vi "FringeTrackerGUI.vi"() -> ()   [LabVIEW 2009, in "FringeTracker.lvlib"]
uses:
  FringeTracker.lvlib
  Controls/FringeTrackerInfo.ctl
  Nicmos/Controls/NICMOS.READOUT.ctl
  Controls/FringeTrackerData.ctl
panel:
  in  "Autcollimation":bool
  in  "Wavelength":dbl[unit]
  in  "Readout":T1
  out "FringeTrackerInfo":T2={"Readout"={"Readout"=100, "Deglitch"=10, "Framerate"=200.0, "Bank"=2}, "OPD stroke"=0.0, "OPD per pixel"=0.0}
  in  "IDLE Button":bool
  in  "SCAN Button":bool
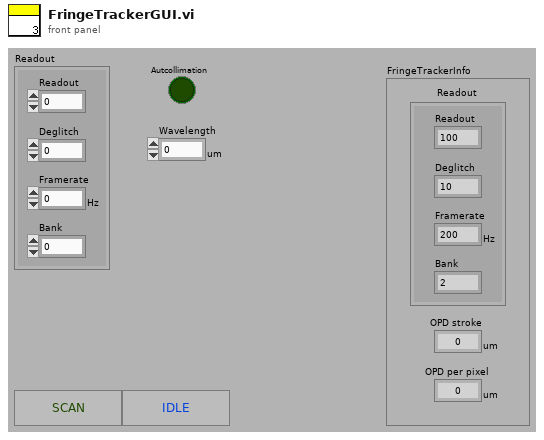
[diagram p1: front panel]
types:
  T1 = typedef "NICMOS.READOUT.ctl" = cluster{"Readout":i32, "Deglitch":i32, "Framerate":dbl[unit], "Bank":i32}
  T2 = typedef "FringeTrackerInfo.ctl" = cluster{"Readout":T1, "OPD stroke":dbl[unit], "OPD per pixel":dbl[unit]}
  T3 = typedef "FringeTrackerData.ctl" = cluster{"Readout":T1, "Wavelength":dbl[unit], "Frame per fringe":dbl, "Autcollimation":bool, "OPD stroke":dbl[unit], "OPD per pixel":dbl[unit], "Offset":dbl[unit]}
  T4 = typedef "FringeTrackerState.ctl" = enum16{"IDLING", "CONFIGURING", "SCANNING", "SEARCHING", "TRACKING", "STOPPING"}
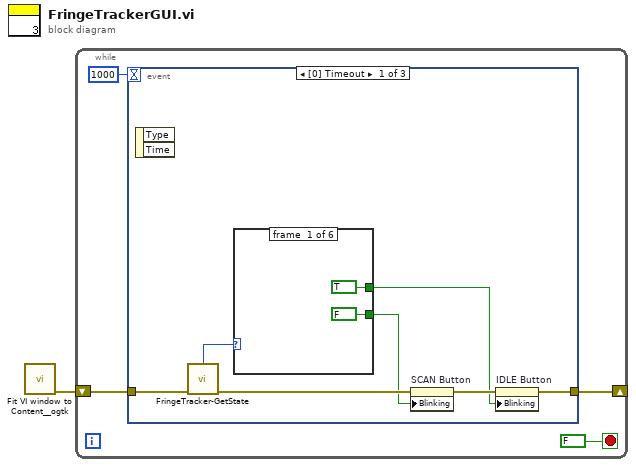
[diagram p0: block diagram]
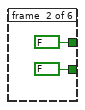
[diagram p2: hidden frame]
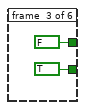
[diagram p3: hidden frame]
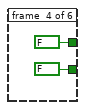
[diagram p4: hidden frame]
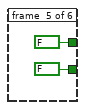
[diagram p5: hidden frame]
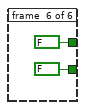
[diagram p6: hidden frame]
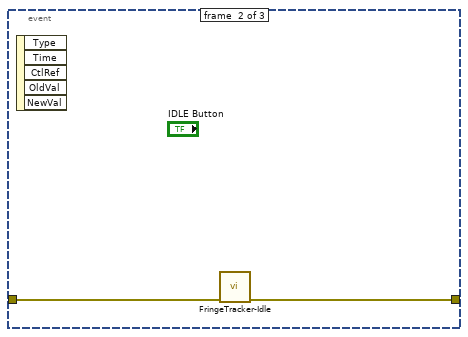
[diagram p7: hidden frame]
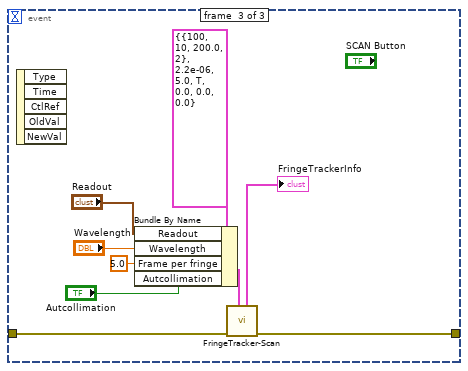
[diagram p8: hidden frame]
diagram:
  n1 = call <userlib>:"Fit VI window to Content__ogtk.vi"() -> ("error out"=w1:errorcluster)  [unwired: 6 in, 1 out]
  n2 = while {
    shift-right: [w4] -> _
    shift-left: w1 -> [w5]
    stop <- FALSE stop-if-true
    n3 = event shown="[0] Timeout" {
      selector: _ -> [_ _ _]
      dyn-events: _ -> [_ _ _]
      timeout: 1000 -> [_ _ _]
      tunnel: w5 -> [w12 w26 w35]
      tunnel: [w8 w25 w34] -> w4
      event #0 {
        n4 = event-data() -> ()  [unwired: 1 in, 2 out]
        n5 = call "FringeTracker-GetState.vi"("error in (no error)"=w12) -> ("State"=w11:T4, "error out"=w9:errorcluster)  [unwired: 7 in]
        n6 = case shown="\"IDLING\", Default" w11 {
          tunnel: [TRUE FALSE FALSE FALSE FALSE FALSE] -> w7
          tunnel: [FALSE FALSE TRUE FALSE FALSE FALSE] -> w6
          frame #0 {
          }
          frame #1 {
          }
          frame #2 {
          }
          frame #3 {
          }
          frame #4 {
          }
          frame #5 {
          }
        }
        n7 = property on="SCAN Button" class="Bool"(error in=w9, "Blinking"=w6) -> (error out=w10:errorcluster)  [unwired: 1 in, 1 out]
        n8 = property on="IDLE Button" class="Bool"(error in=w10, "Blinking"=w7) -> (error out=w8:errorcluster)  [unwired: 1 in, 1 out]
      }
      event #1 {
        n9 = event-data() -> ()  [unwired: 1 in, 5 out]
        n10 = call "FringeTracker-Idle.vi"("error in (no error)"=w26) -> ("error out"=w25:errorcluster)  [unwired: 10 in]
      }
      event #2 {
        n11 = event-data() -> ()  [unwired: 1 in, 5 out]
        n12 = Bundle By Name(cluster=T3 {"Readout"={"Readout"=100, "Deglitch"=10, "Framerate"=200.0, "Bank"=2}, "Wavelength"=2.2e-06, "Frame per fringe"=5.0, "Autcollimation"=TRUE, "OPD stroke"=0.0, "OPD per pixel"=0.0, "Offset"=0.0} ("FringeTrackerData"), "Readout"="Readout", "Wavelength"="Wavelength", "Frame per fringe"=5.0, "Autcollimation"="Autcollimation") -> (w31:T3)
        n13 = call "FringeTracker-Scan.vi"("FringeTrackerData"=w31, "error in (no error)"=w35) -> ("error out"=w34:errorcluster, "FringeTrackerInfo"=→"FringeTrackerInfo":T2)  [unwired: 8 in]
      }
    }
  }
